vi "Clenshaw2.vi"(10 "c":dbl[](array[numeric]), 11 "x":dbl[](array[numeric])) -> (3 "y":dbl[](array[numeric]))   [LabVIEW 2019]
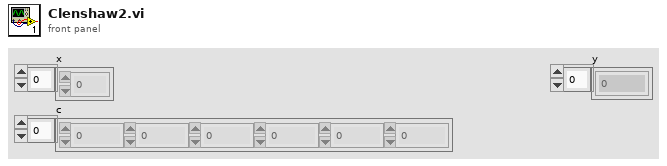
[diagram p1: front panel]
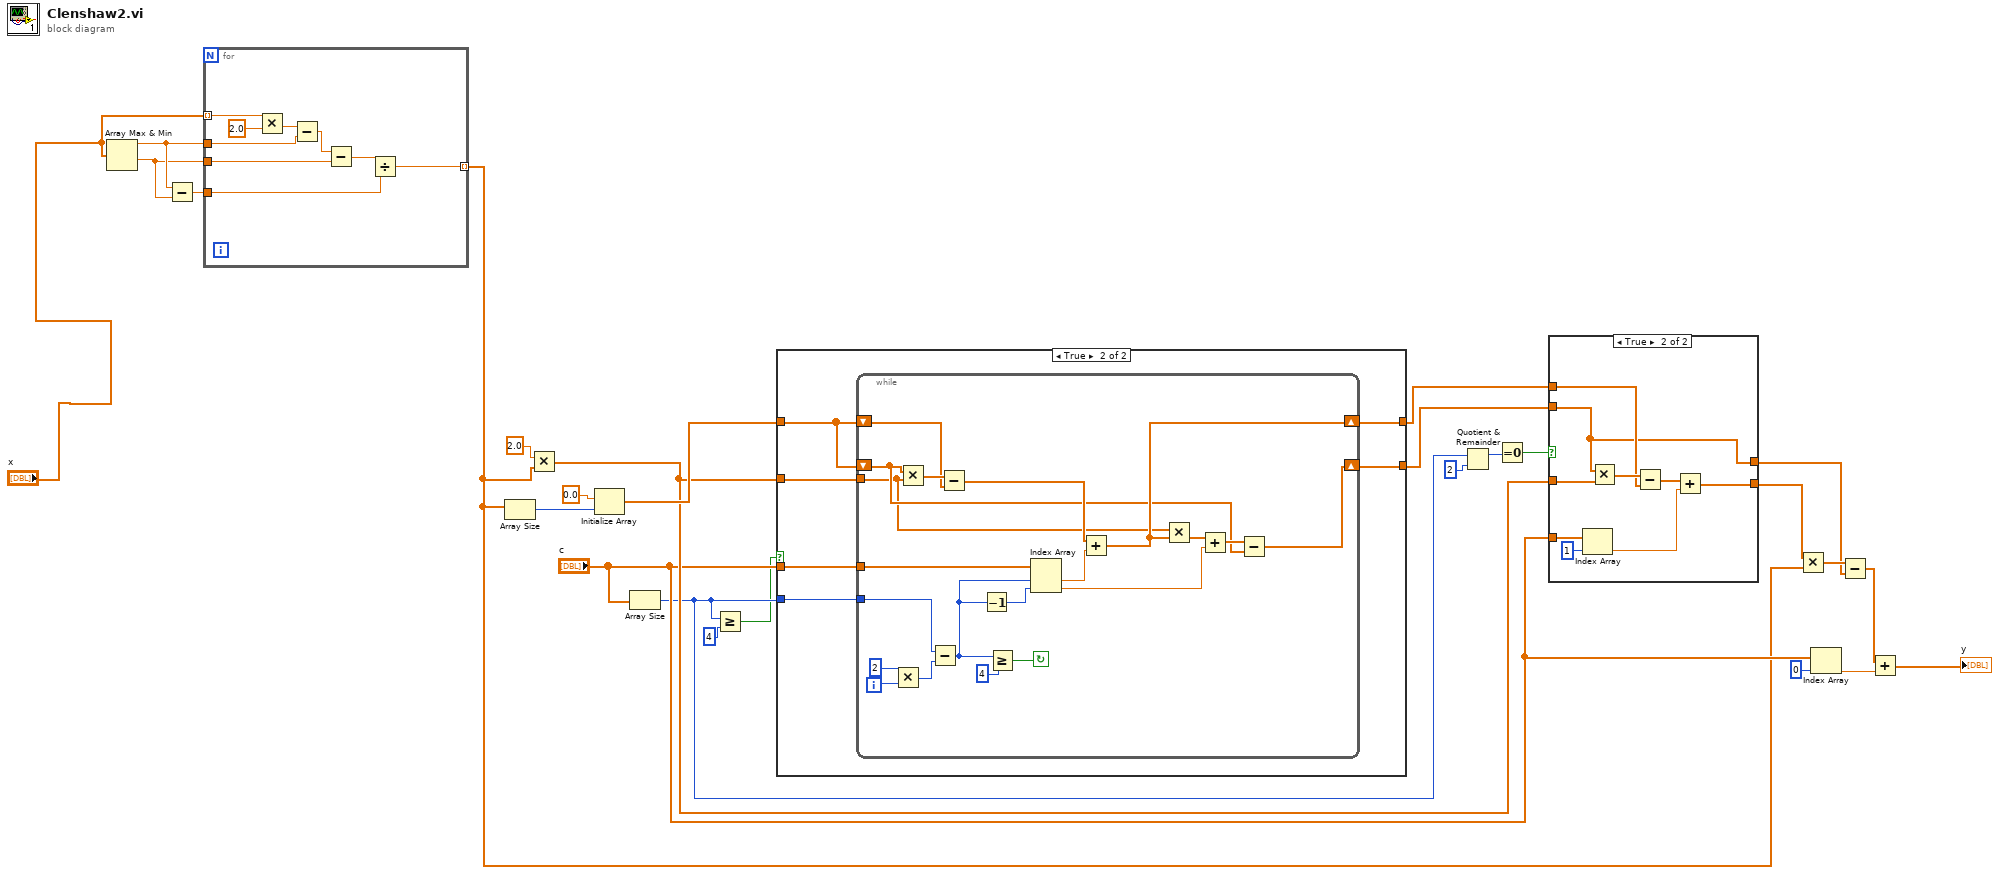
[diagram p0: block diagram]
diagram:
  n1 = Array Max & Min(array="x") -> (max value=w6:dbl, min value=w5:dbl)  [unwired: 2 out]
  n2 = Subtract(x=w6, y=w5) -> (x-y=w4:dbl)
  n3 = for {
    tunnel: "x" -> [w35] mode=indexing
    tunnel: w6 -> [w32]
    tunnel: w5 -> [w30]
    tunnel: w4 -> [w28]
    tunnel: [w27] -> w1 mode=indexing
    n4 = Multiply(x=w35, y=2.0) -> (x*y=w33:dbl)
    n5 = Subtract(x=w33, y=w32) -> (x-y=w31:dbl)
    n6 = Subtract(x=w31, y=w30) -> (x-y=w29:dbl)
    n7 = Divide(x=w29, y=w28) -> (x/y=w27:dbl)
  }
  n8 = Array Size(array=w1) -> (size(s)=w26:i32)
  n9 = Multiply(x=2.0 ("element"), y=w1) -> (x*y=w17:dbl[])
  n10 = Initialize Array(0.0 ("element"), w26) -> (w23:dbl[])
  n11 = Array Size(array="c") -> (size(s)=w9:i32)
  n12 = Greater Or Equal?(x=w9, y=4) -> (x >= y?=w7:bool)
  n13 = case shown="True" w7 {
    tunnel: w23 -> [w36 w37]
    tunnel: w9 -> [_ w42]
    tunnel: [w36 w41] -> w19
    tunnel: [w36 w40] -> w18
    tunnel: w17 -> [_ w39]
    tunnel: "c" -> [_ w38]
    frame False {
    }
    frame True {
      n14 = while {
        shift-right: [w49] -> w41
        shift-left: w37 -> [w54]
        shift-right: [w50] -> w40
        shift-left: w37 -> [w48]
        tunnel: w38 -> [w45]
        tunnel: w42 -> [w44]
        tunnel: w39 -> [w43]
        i -> [w62]
        stop <- w57 continue-if-true
        n15 = Multiply(x=2, y=w62) -> (x*y=w56:i32)
        n16 = Multiply(x=w48, y=w43) -> (x*y=w55:dbl[])
        n17 = Subtract(x=w44, y=w56) -> (x-y=w58:i32)
        n18 = Subtract(x=w55, y=w54) -> (x-y=w51:dbl[])
        n19 = Decrement(x=w58) -> (x-1=w59:i32)
        n20 = Greater Or Equal?(x=w58, y=4) -> (x >= y?=w57:bool)
        n21 = Index Array(array=w45, index #1=w58, index #2=w59) -> (element #1=w47:dbl, element #2=w46:dbl)
        n22 = Add(x=w51, y=w47) -> (x+y=w49:dbl[])
        n23 = Multiply(x=w43, y=w49) -> (x*y=w53:dbl[])
        n24 = Add(x=w53, y=w46) -> (x+y=w52:dbl[])
        n25 = Subtract(x=w52, y=w48) -> (x-y=w50:dbl[])
      }
    }
  }
  n26 = Quotient & Remainder(x=w9, y=2) -> (x-y*floor(x/y)=w21:i32)  [unwired: 1 out]
  n27 = Equal To 0?(x=w21) -> (x = 0?=w20:bool)
  n28 = case shown="True" w20 {
    tunnel: w19 -> [w64 w69]
    tunnel: w18 -> [w63 w65]
    tunnel: "c" -> [_ w73]
    tunnel: w17 -> [_ w71]
    tunnel: [w63 w66] -> w13
    tunnel: [w64 w65] -> w11
    frame False {
    }
    frame True {
      n29 = Index Array(array=w73, index=1) -> (element=w67:dbl)
      n30 = Multiply(x=w65, y=w71) -> (x*y=w70:dbl[])
      n31 = Subtract(x=w70, y=w69) -> (x-y=w68:dbl[])
      n32 = Add(x=w68, y=w67) -> (x+y=w66:dbl[])
    }
  }
  n33 = Multiply(x=w13, y=w1) -> (x*y=w12:dbl[])
  n34 = Index Array(array="c", index=0) -> (element=w14:dbl)
  n35 = Subtract(x=w12, y=w11) -> (x-y=w10:dbl[])
  n36 = Add(x=w10, y=w14) -> (x+y=→"y":dbl[])
